vi "Process VIA.vi"(8 "error in (no error)":errorcluster, 10 "Raw VIA":string, 11 "DeployTarget in":refnum<class "Platform.lvclass">) -> (0 "error out":errorcluster, 2 "VIA":string, 3 "DeployTarget out":refnum<class "Platform.lvclass">)   [LabVIEW 2020, in "PicoG-Core.lvlib" / "Platform.lvclass"]
uses:
  Platform.lvclass
  Platform.lvclass/Platform.ctl
  PicoG-Core.lvlib
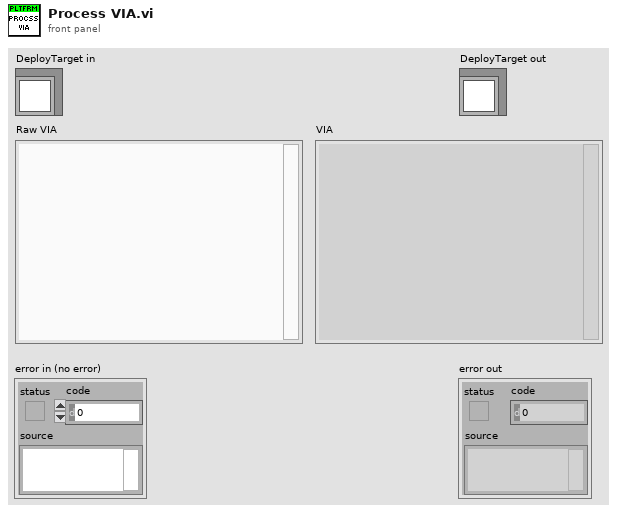
[diagram p1: front panel]
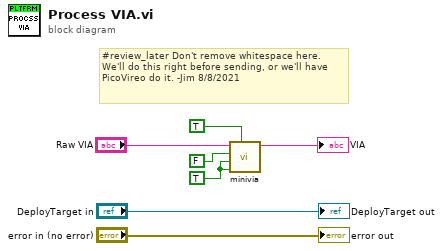
[diagram p0: block diagram]
diagram:
  w1 = TRUE ("Remove Whitespace")
  # "#review_later Don't remove whitespace here. We'll do this right before sending, or we'll have PicoVireo do it. -Jim 8/8/2021"
  n1 = call "minivia.vi"("Minify Locals?"=TRUE, "Remove Enqueue?"=w1, "Remove JavaScriptInvoke"=w1, "Remove Whitespace"=FALSE, "VIA"="Raw VIA") -> ("Minified"=→"VIA":string)  [unwired: 6 in]
  "error out" <- "error in (no error)"
  "DeployTarget out" <- "DeployTarget in"
